vi "BinaryTOBCDconverter.vi"() -> ()   [LabVIEW 2018]
panel:
  out "B 8":bool
  out "B 7":bool
  out "B 6":bool
  out "B 5":bool
  out "B 4":bool
  out "B 3":bool
  out "B 2":bool
  out "B1":bool
  in  "A5":bool
  in  "A4":bool
  in  "A3":bool
  in  "A2":bool
  in  "A1":bool
  in  "A0":bool
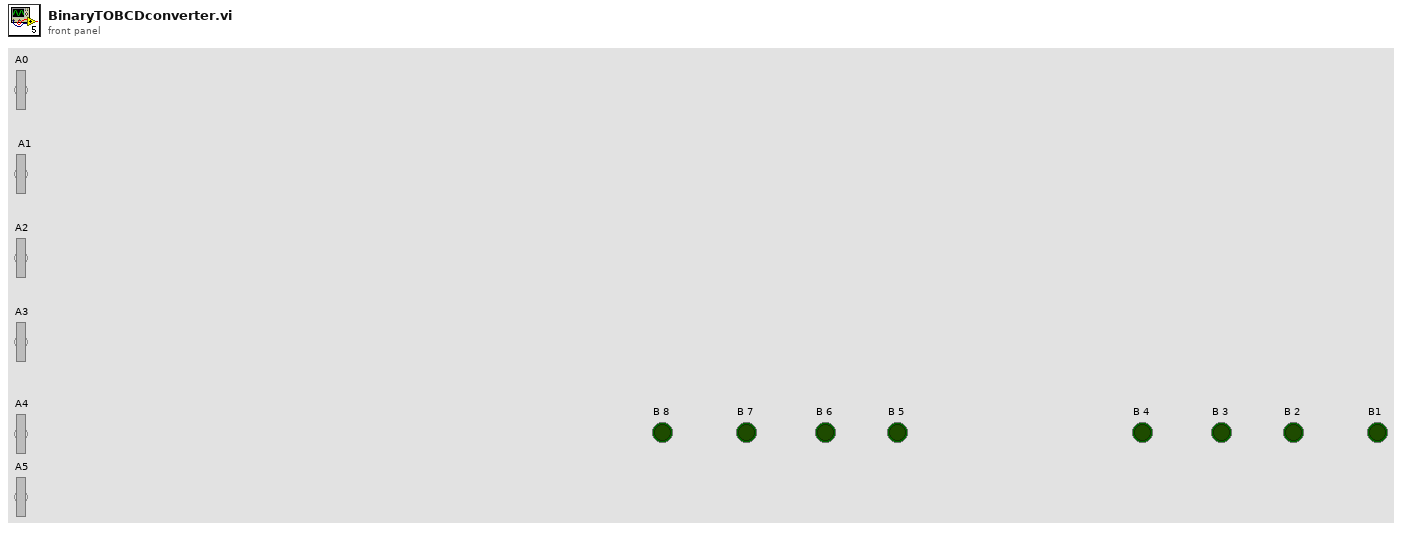
[diagram p1: front panel]
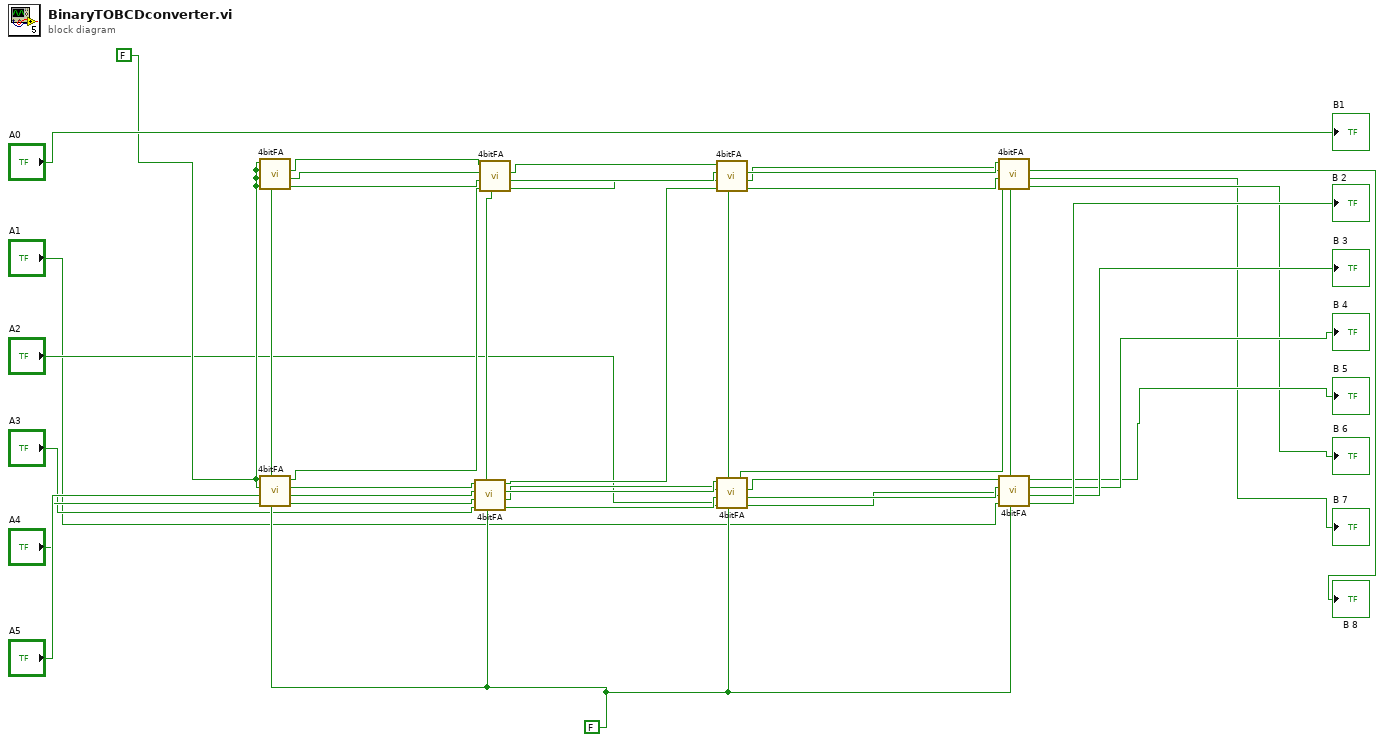
[diagram p0: block diagram]
diagram:
  w11 = FALSE
  w36 = FALSE
  n1 = call "4bitFA.vi"("Cin"=w36, "A1"="A4", "A2"="A5", "A4"=w11, "A8"=w11) -> ("B2"=w33:bool, "B4"=w34:bool, "B8"=w35:bool, "B1"=w17:bool, "Cout"=w40:bool)
  n2 = call "4bitFA.vi"("Cin"=w40, "A1"=w11, "A2"=w11, "A4"=w11, "A8"=w11) -> ("B2"=w24:bool, "B4"=w25:bool, "B8"=w26:bool)  [unwired: 2 out]
  n3 = call "4bitFA.vi"("Cin"=w36, "A1"="A3", "A2"=w33, "A4"=w34, "A8"=w35) -> ("B2"=w30:bool, "B4"=w31:bool, "B8"=w32:bool, "B1"=w16:bool, "Cout"=w39:bool)
  n4 = call "4bitFA.vi"("Cin"=w39, "A1"=w17, "A2"=w24, "A4"=w25, "A8"=w26) -> ("B2"=w21:bool, "B4"=w22:bool, "B8"=w23:bool)  [unwired: 2 out]
  n5 = call "4bitFA.vi"("Cin"=w36, "A1"="A2", "A2"=w30, "A4"=w31, "A8"=w32) -> ("B2"=w27:bool, "B4"=w28:bool, "B8"=w29:bool, "B1"=w15:bool, "Cout"=w38:bool)
  n6 = call "4bitFA.vi"("Cin"=w38, "A1"=w16, "A2"=w21, "A4"=w22, "A8"=w23) -> ("B2"=w18:bool, "B4"=w19:bool, "B8"=w20:bool)  [unwired: 2 out]
  n7 = call "4bitFA.vi"("Cin"=w36, "A1"="A1", "A2"=w27, "A4"=w28, "A8"=w29) -> ("B2"=→"B 2":bool, "B4"=→"B 3":bool, "B8"=→"B 4":bool, "B1"=→"B 5":bool, "Cout"=w37:bool)
  n8 = call "4bitFA.vi"("Cin"=w37, "A1"=w15, "A2"=w18, "A4"=w19, "A8"=w20) -> ("B2"=→"B 6":bool, "B4"=→"B 7":bool, "B8"=→"B 8":bool)  [unwired: 2 out]
  "B1" <- "A0"
